vi "TAI_Motor.vi"(3 "Normal Output":dbl, 4 "Override Actuator Bypass":bool, 5 "Actuator Name":string) -> (0 "Interlocked Output":dbl, 2 "Output Mode":T1(ring))   [LabVIEW 2020]
doc: "This VI is configured for polymorphic use and functions as an interlock, allowing the selected motor to be tested manually via the FRC 4265 Dashboard. During testing, all interlocked actuators which are not selected for testing are disabled."
uses:
  b41506b6-27dc-4ca7-820b-83b05fbff20d.vi
  ce8c15ce-250d-419c-a833-6f2ecce11d20.vi
  driverdata.vi
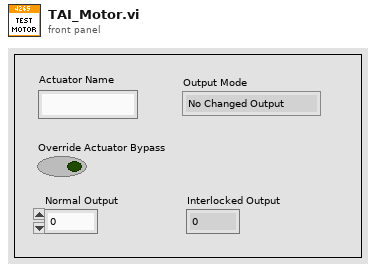
[diagram p1: front panel]
types:
  T1 = enum16{"No Changed Output", "New Normal Output", "New Testing Output"}
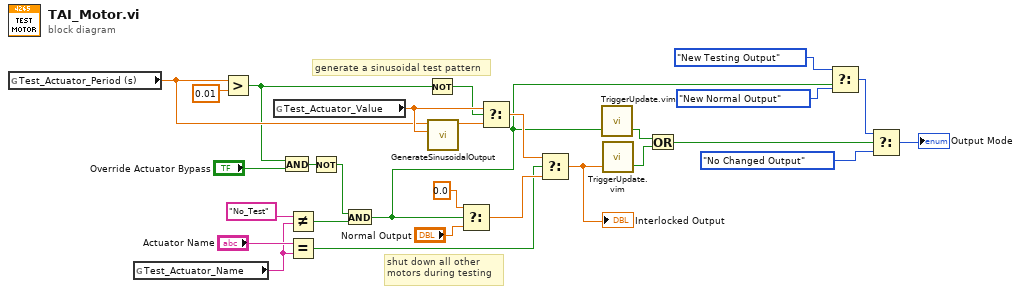
[diagram p0: block diagram]
diagram:
  # "generate a sinusoidal test pattern"
  # "shut down all other\nmotors during testing"
  n1 = global read "driverdata.vi" "Test_Actuator_Period (s)"() -> (w19:dbl)
  n2 = global read "driverdata.vi" "Test_Actuator_Name"() -> (w23:string)
  n3 = Greater?(x=w19, y=0.01) -> (0:w15:bool)
  n4 = global read "driverdata.vi" "Test_Actuator_Value"() -> (w20:dbl)
  n5 = And(x=w15, y="Override Actuator Bypass") -> (x .and. y?=w13:bool)
  n6 = Not Equal?(x="No_Test", y=w23) -> (x != y?=w17:bool)
  n7 = Equal?(x="Actuator Name", y=w23) -> (x = y?=w5:bool)
  n8 = Not(x=w13) -> (.not. x?=w16:bool)
  n9 = And(x=w16, y=w17) -> (x .and. y?=w1:bool)
  n10 = Not(x=w15) -> (.not. x?=w12:bool)
  n11 = call "GenerateSinusoidalOutput.vi"("Amplitude"=w20, "Period (s)"=w19) -> ("sin(time)"=w22:dbl)  [unwired: 9 in]
  n12 = Select(t=0.0, s=w1, f="Normal Output") -> (s? t:f=w24:dbl)
  n13 = Select(t=w20, s=w12, f=w22) -> (s? t:f=w21:dbl)
  n14 = Select(t=w21, s=w5, f=w24) -> (s? t:f=w11:dbl)
  "Interlocked Output" <- w11
  n15 = call "TriggerUpdate.vim"("Trigger"=w1) -> ("Update"=w4:bool)  [unwired: 2 in]
  n16 = call "TriggerUpdate.vim"("Trigger"=w11) -> ("Update"=w3:bool)  [unwired: 2 in]
  n17 = Or(x=w4, y=w3) -> (x .or. y?=w2:bool)
  n18 = Select(t=T1."New Testing Output", s=w1, f=T1."New Normal Output") -> (s? t:f=w8:T1)
  n19 = Select(t=w8, s=w2, f=T1."No Changed Output") -> (s? t:f=→"Output Mode":T1)
